vi "BubbleSortUsingInplaceElementStructure.vi"(0 "Input Array":dbl[](array[numeric])=[5.0, 4.0, 3.0, 2.0, 1.0, 0.0], 5 "Sorting Type":T1) -> (4 "Output Array":dbl[](array[numeric]))   [LabVIEW 2020]
uses:
  Typedefs/SortType.ctl
panel:
  in  "Stop":bool
  # "Sorting of Arrays"
  # "Description:\n1. Add the array that has to be sorted in the input array. \n2. Then select the appropriate sorting to be done. \n3.  Once selected the output will be displayed in the Output Array.\n4. Press stop to stop the whole process."
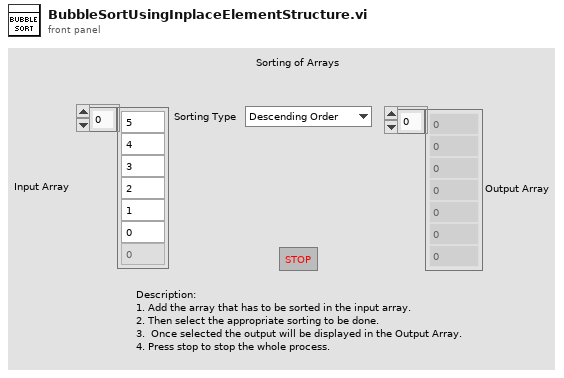
[diagram p1: front panel]
types:
  T1 = typedef "SortType.ctl" = enum16{"Descending Order", "Ascending Order"}
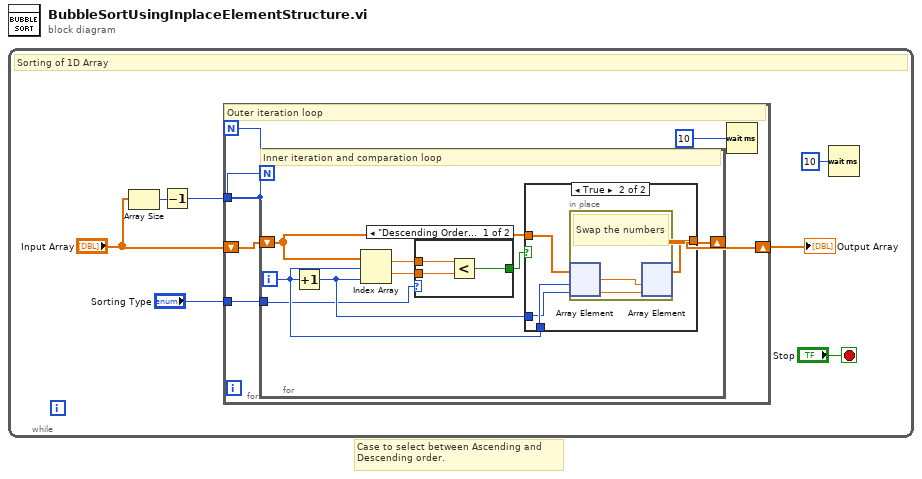
[diagram p0: block diagram]
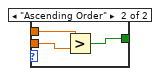
[diagram p2: hidden frame]
diagram:
  # "Case to select between Ascending and \nDescending order."
  n1 = while {
    stop <- "Stop" stop-if-true
    # "Sorting of 1D Array"
    n2 = Array Size(array="Input Array") -> (size(s)=w6:i32)
    n3 = Decrement(x=w6) -> (x-1=w5:i32)
    n4 = for {
      N: w5 -> [_]
      shift-right: [w10] -> w4
      shift-left: "Input Array" -> [w12]
      tunnel: w5 -> [w11]
      tunnel: "Sorting Type" -> [w8]
      # "Outer iteration loop"
      n5 = for {
        N: w11 -> [_]
        shift-right: [w18] -> w10
        shift-left: w12 -> [w20]
        tunnel: w8 -> [w13]
        i -> [w19]
        # "Inner iteration and comparation loop"
        n6 = Increment(x=w19) -> (x+1=w14:i32)
        n7 = Index Array(array=w20, index #1=w19, index #2=w14) -> (element #1=w16:dbl, element #2=w15:dbl)
        n8 = case shown="\"Descending Order\", Default" w13 {
          tunnel: w16 -> [w22 w25]
          tunnel: w15 -> [w21 w24]
          tunnel: [w23 w26] -> w17
          frame "Descending Order", Default {
            n9 = Less?(x=w22, y=w21) -> (x < y?=w23:bool)
          }
          frame "Ascending Order" {
            n10 = Greater?(x=w25, y=w24) -> (0:w26:bool)
          }
        }
        n11 = case shown="True" w17 {
          tunnel: w20 -> [w27 w28]
          tunnel: w19 -> [_ w31]
          tunnel: [w27 w29] -> w18
          tunnel: w14 -> [_ w30]
          frame False {
          }
          frame True {
            n12 = in-place {
              # "Swap the numbers"
              n13 = in-place-array #1(w28, w31, w30) -> (w32:dbl, w33:dbl)
              n14 = in-place-array #1(w33, w32) -> (w29:dbl[])  [unwired: 2 out]
            }
          }
        }
      }
      n15 = Wait (ms)(milliseconds to wait=u32 10) -> ()  [unwired: 1 out]
    }
    "Output Array" <- w4
    n16 = Wait (ms)(milliseconds to wait=u32 10) -> ()  [unwired: 1 out]
  }
